vi "Read Spectral Waveform.vi"(8 "error in (no error)":errorcluster, 11 "VISA resource name":refnum<visa-resource-name>) -> (0 "error out":errorcluster, 2 "Spectral Waveform":T1(graph), 3 "VISA resource name out":refnum<visa-resource-name>)   [LabVIEW 2015, in "Micron Optics sm130.lvlib"]
doc: "Displays the spectral data in a waveform for the selected channel in Configure Channel.vi."
uses:
  Micron Optics sm130.lvlib
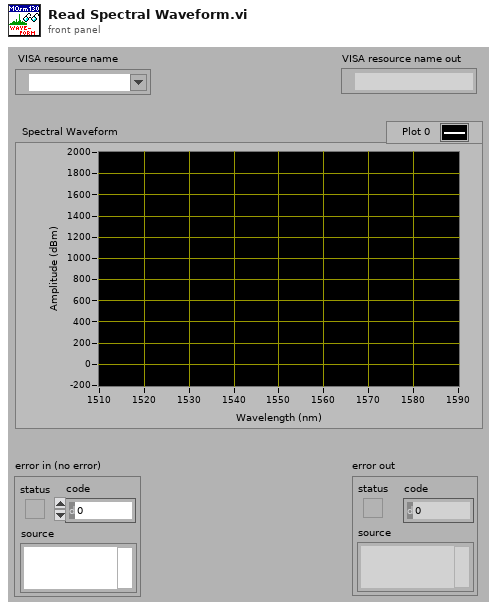
[diagram p1: front panel]
types:
  T1 = cluster{"Wavelength (nm)":dbl[], "Spectrum":i16[]}[]
  T2 = cluster{"Wavelength (nm)":dbl[], "Spectra":i16[]}
  T3 = cluster{"Wavelength (nm)":dbl[], "Spectra":i16[]}[]
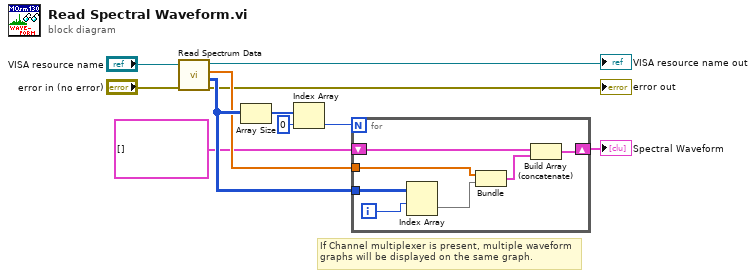
[diagram p0: block diagram]
diagram:
  # "If Channel multiplexer is present, multiple waveform graphs will be displayed on the same graph."
  n1 = call "Read Spectrum Data.vi"("error in (no error)"="error in (no error)", "VISA resource name"="VISA resource name") -> ("error out"=→"error out":errorcluster, "Spectra"=w9:i16[][], "Wavelength (nm)"=w8:dbl[], "VISA resource name out"=→"VISA resource name out":refnum<visa-resource-name>)  [unwired: 5 in, 1 out]
  n2 = Array Size(array=w9) -> (size(s)=w3:i32[])
  n3 = Index Array(array=w3, index=0) -> (element=w1:i32)
  n4 = for {
    N: w1 -> [_]
    tunnel: w9 -> [w15]
    tunnel: w8 -> [w18]
    shift-right: [w16] -> w6
    shift-left: T1 [] -> [w17]
    i -> [w12]
    n5 = Index Array(array=w15, index (row)=w12) -> (element=w14:i16[])  [unwired: 1 in]
    n6 = Bundle("Wavelength (nm)"=w18, "Spectra"=w14) -> (w13:T2)  [unwired: 1 in]
    n7 = Build Array (concatenate)(w17, w13) -> (w16:T3)
  }
  "Spectral Waveform" <- w6
